vi "TEST.vi"() -> ()   [LabVIEW 2011]
uses:
  TCPIPconfig.ctl
  TCPIP_enum.ctl
panel:
  out "error out":errorcluster
  out "LED":bool[](array[boolean])
  in  "config":T1=[{"add"="192.168.0.69", "port"=6340, "timeout"=800, "connection ID"=refnum, "targer"=enum."主舱外回路"}]
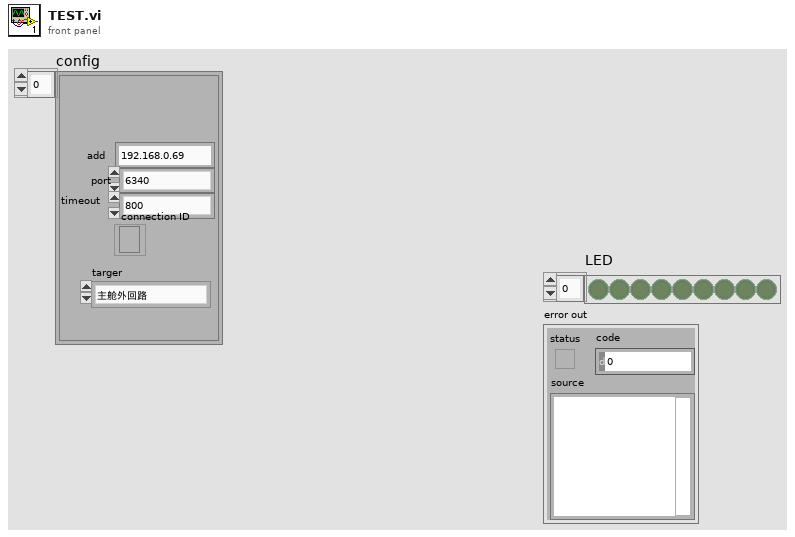
[diagram p1: front panel]
types:
  T1 = typedef "TCPIPconfig.ctl" = cluster{"add":string, "port":u32, "timeout":u16, "connection ID":refnum<k5>, "targer":enum16{"主舱外回路", "主舱内回路", "实验舱外回路", "实验舱内回路"}}[]
  T2 = typedef "TCPIP_enum.ctl" = enum16{"init", "connect", "command", "write", "read", "close", "null"}
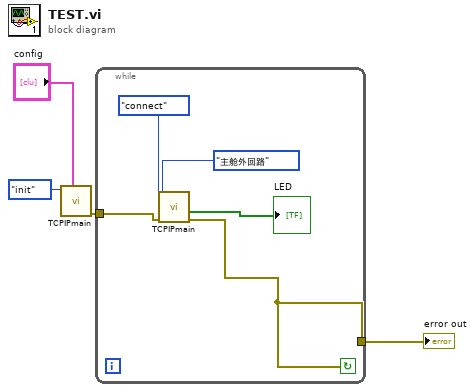
[diagram p0: block diagram]
diagram:
  n1 = call "TCPIPmain.vi"("config"="config", "Enum"=TCPIP_enum."init") -> ("error out"=w2:errorcluster)  [unwired: 7 in, 2 out]
  n2 = while {
    tunnel: w2 -> [w9]
    tunnel: [w5] -> w1
    stop <- w5 continue-if-true
    n3 = call "TCPIPmain.vi"("error in"=w9, "targer"=enum16{"主舱外回路", "主舱内回路", "实验舱外回路", "实验舱内回路"}."主舱外回路", "Enum"=TCPIP_enum."connect") -> ("error out"=w5:errorcluster, "LED"=→"LED":bool[])  [unwired: 6 in, 1 out]
  }
  "error out" <- w1
